vi "WSS Modes to Word.vi"(11 "Wheel Speed Sensor Modes":T1) -> (3 "Wheel Speed Sensor Word":u16)   [LabVIEW 2014, in "SLSC configuration Shared.lvlib"]
doc: "Converts four faults to a fault word."
uses:
  SLSC configuration Shared.lvlib
  WSS Mode Array.ctl
  WSS Mode.ctl
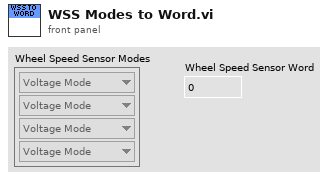
[diagram p1: front panel]
types:
  T1 = typedef "SLSC configuration Shared.lvlib/WSS Mode Array.ctl" = T2[]
  T2 = typedef "SLSC configuration Shared.lvlib/WSS Mode.ctl" = enum8{"Voltage Mode", "Current Mode"}
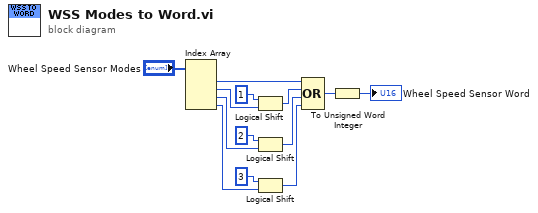
[diagram p0: block diagram]
diagram:
  n1 = Index Array(array="Wheel Speed Sensor Modes") -> (element #1=w9:T2, element #2=w6:T2, element #3=w3:T2, element #4=w1:T2)  [unwired: 4 in]
  n2 = Logical Shift(y=u16 1, x=w6) -> (x << y=w10:u32)
  n3 = Logical Shift(y=u16 2, x=w3) -> (x << y=w11:u32)
  n4 = Logical Shift(y=i16 3, x=w1) -> (x << y=w7:u32)
  n5 = Compound Arithmetic op=OR(w9, w10, w11, w7) -> (w12:u32)
  n6 = To Unsigned Word Integer(number=w12) -> (unsigned 16bit integer=→"Wheel Speed Sensor Word":u16)
